vi "us read.vi"(8 "Error In":errorcluster, 11 "my FPGA lib.lvlib:US sensor.lvclass":refnum<class "US sensor.lvclass">) -> (0 "error out":errorcluster, 1 "DC estimate (V)":dbl format="%0.2f", 2 "AC estimate (Vrms)":dbl format="%0.2f", 3 "my FPGA lib.lvlib:US sensor.lvclass 2":refnum<class "US sensor.lvclass">, 4 "s? t:f":dbl)   [LabVIEW 2019]
uses:
  FPGA_subVIs/low level/us sensor/US sensor.lvclass
  <vilib>/ptbypt/NI_PtbyPt.lvlib
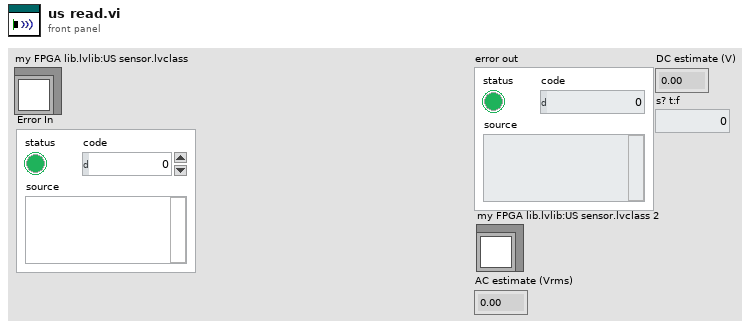
[diagram p1: front panel]
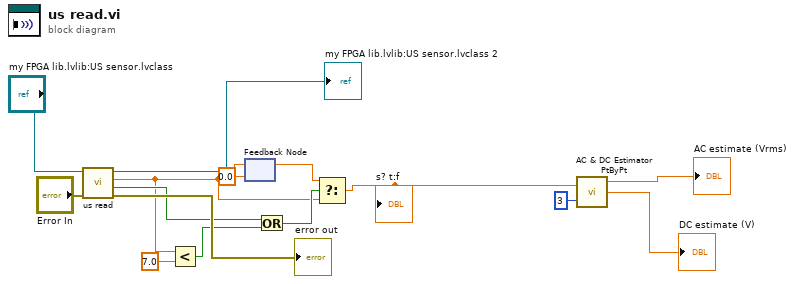
[diagram p0: block diagram]
diagram:
  n1 = call "us read.vi"("Error In"="Error In", "my FPGA lib.lvlib:US sensor.lvclass"="my FPGA lib.lvlib:US sensor.lvclass") -> ("error out"=→"error out":errorcluster, "timeout?"=w5:bool, "distance(cm)"=w3:dbl, "my FPGA lib.lvlib:US sensor.lvclass 2"=→"my FPGA lib.lvlib:US sensor.lvclass 2":refnum<class "US sensor.lvclass">)  [unwired: 6 in]
  n2 = Less?(x=w3, y=7.0) -> (x < y?=w1:bool)
  n3 = feedback-in #1(w3) -> ()
  n4 = feedback #1(0.0 ("distance(cm)")) -> (w10:dbl)
  n5 = Or(x=w5, y=w1) -> (x .or. y?=w4:bool)
  n6 = Select(t=w10, s=w4, f=w3) -> (s? t:f=w6:dbl)
  "s? t:f" <- w6
  n7 = call <vilib>:"AC & DC Estimator PtByPt.vi"("signal"=w6, "sample length"=3) -> ("AC estimate (Vrms)"=→"AC estimate (Vrms)":dbl, "DC estimate (V)"=→"DC estimate (V)":dbl)  [unwired: 1 in, 1 out]
